vi "cs-scanning_v5_refsonly.vi"() -> ()   [LabVIEW 2017]
uses:
  controls/boolean_info.ctl
  controls/TF-params.ctl
  controls/z-axis-params_v4.ctl
  <vilib>/rvi/Emulation/niFpgaGetClockAttributes.vi
  <vilib>/rvi/Emulation/niFpgaSctlEmulationGetInTimedLoop.vi
  <vilib>/rvi/Emulation/niFpgaEmulationReportErrorSimple.vi
  <vilib>/rvi/Emulation/niFpgaProcessEmulError.vi
  <vilib>/rvi/eio/common/nirviEmuTemplateMethod_errors.vi
  <vilib>/rvi/Emulation/niFpgaEmulationIsFPGAContextNoSignature.vi
  <vilib>/rvi/DataTransferAndStorage/Container/Common/niFpgaContainerGetUniqueNameForEmu.vi
  <vilib>/rvi/Memory/Memory_Emulation/niFpgaMemoryEmulationCacheClearOnFirstRun.vi
  <vilib>/rvi/Memory/Memory_Emulation/nirvimemoryEmulationManagerCache_MakeExclusive.vi
  <vilib>/rvi/Memory/Memory_Emulation/niFpgaMemoryEmulationValidateCache.vi
  <vilib>/rvi/Memory/Memory_Emulation/nirvimemoryEmulationManagerCache_InsertValue.vi
  <vilib>/Utility/error.llb/Clear Errors.vi
  <vilib>/rvi/Memory/Memory_Emulation/nirvimemoryEmulationManagerCache_ReleaseExclusive.vi
  <vilib>/rvi/Memory/Memory_Emulation/nirvimemoryEmulationManagerCache_GetValue.vi
  <vilib>/rvi/Memory/Memory_Emulation/nirvimemoryEmulationManagerCache_SetValue.vi
  <vilib>/rvi/Emulation/niFpgaCriticalErrorInLSC.vi
  <vilib>/eio/EIONode/EIONode.xnode
  <vilib>/rvi/DataTransferAndStorage/Container/XNode/niFpgaContainer.xnode
  <vilib>/rvi/DataTransferAndStorage/Register/Emulation/niFpgaRegisterEmulation.vi
  FPGA-data-logging.lvlib
  libimaging-cs.lvlib
panel:
  in  "scan-rate":fxp<+/-,16,5>
  in  "zup-err-threshold":fxp<+,24,5>=0.10000038146972656 format="%#_21g"
  in  "z_axis_params":T1={"TOL"=0.3, "z_u_max"=5.0, "setpoint-scan"=0.0, "Ki-scan"=0.001, "Z_error_threshold"=0.0, "Z_settled_samples_threshold "=0, "uz_safe"=0.0, "Kiz_down"=0.001, "max_Z_settle_samples"=5000, "setpoint-up"=0.0} {"uz_safe" format="%#_13g"; "Z_error_threshold" format="%#_13g"; "TOL" format="%#_13g"}
  in  "TF-params":T2={"TF-order"=0, "Num"=[0.0, 0.0, 0.0, 0.0, 0.0, 0.0, 0.0, 0.0, 0.0], "Den"=[0.0, 0.0, 0.0, 0.0, 0.0, 0.0, 0.0, 0.0, 0.0]}
  in  "do-Dz":bool
  out "stop_loops":bool
  out "xy_k":fxp<+/-,16,5>[](array[numeric])
  out "xy_ref":fxp<+/-,16,5>[](array[numeric])
  out "u_x saturated":bool
  out "u_y saturated":bool
  out "state1-count":u64
  out "state5-count":u64
  out "state4-count":u64
  out "state3-count":u64
  out "state2-count":u64
  in  "collect all":bool
  out "entity-index":i16
  in  "TsTicks":u32=1600
  out "number-settled-samples-Z":i16
  out "Current Case":u8
  out "boolean \nindicators":T3
  out "z-u(k)":sgl
  in  "ABORT":bool
  out "read fifo timeout":bool
  in  "numEntities":i16
  in  "trigger-0":bool
  out "number-settled-samples-y":i16
  out "number-settled-samples-x":i16
  in  "xy-error-threshold":sgl format="%#_13g"
  in  "settled-samples\nthreshold":i16
  in  "Ki-xy":sgl=0.001 format="%#_13g"
  in  "xy-bound":sgl
  # "- If collect all = fasle ,\nwe only collect measurement data.\n- If collect all = true, we collect everything."
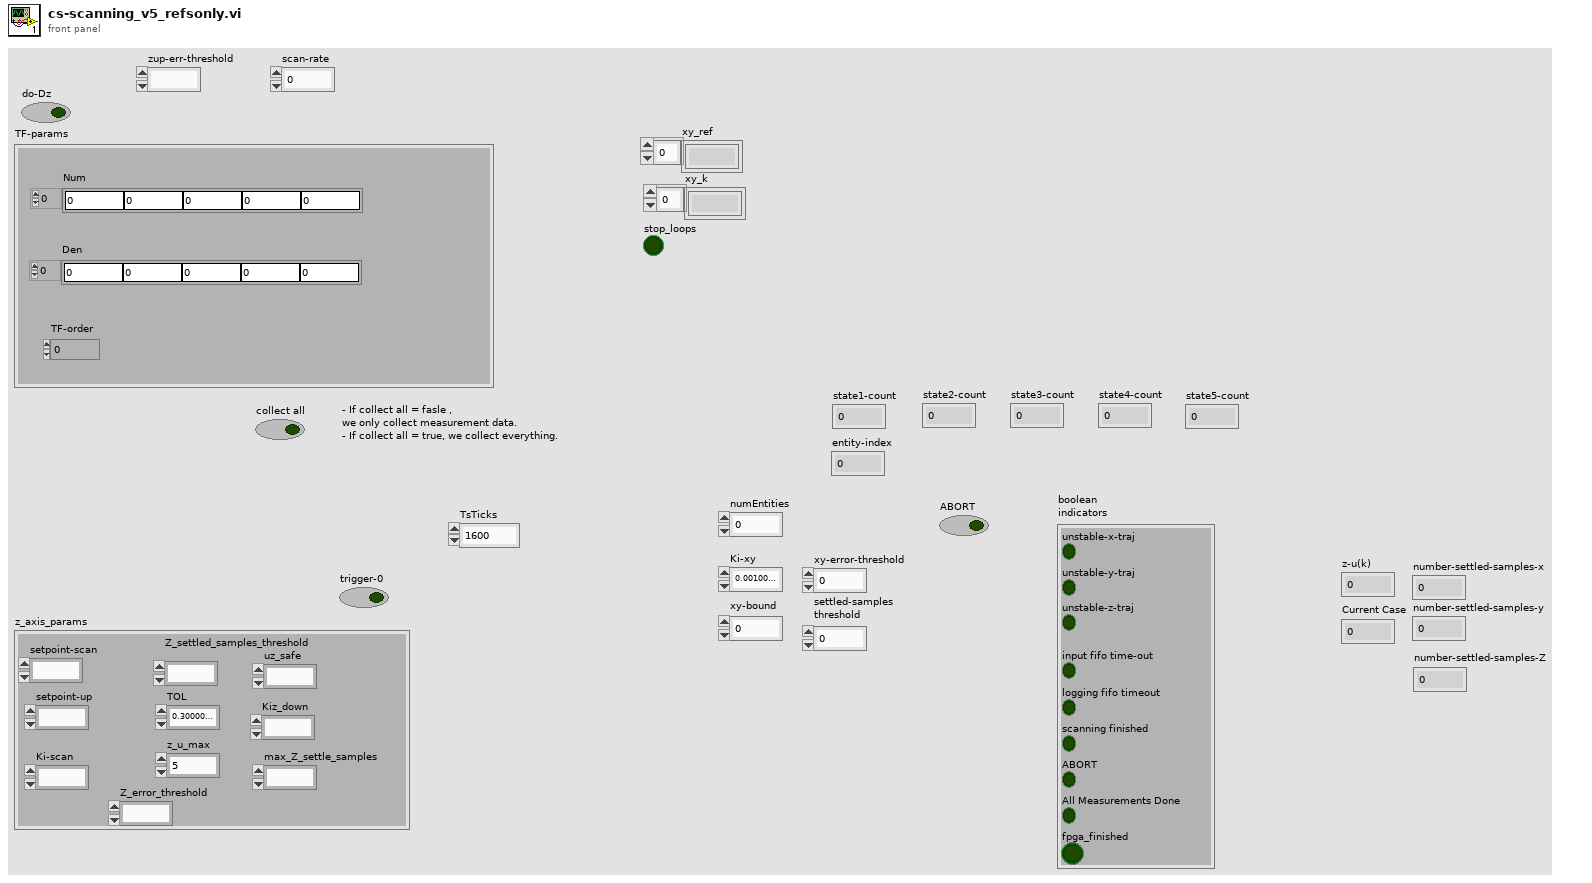
[diagram p1: front panel]
types:
  T1 = typedef "z-axis-params_v4.ctl" = cluster{"TOL":sgl, "z_u_max":sgl, "setpoint-scan":fxp<+/-,32,16>, "Ki-scan":sgl, "Z_error_threshold":sgl, "Z_settled_samples_threshold ":i16, "uz_safe":fxp<+/-,16,5>, "Kiz_down":sgl, "max_Z_settle_samples":i16, "setpoint-up":fxp<+/-,32,16>}
  T2 = typedef "TF-params.ctl" = cluster{"TF-order":i16, "Num":sgl[], "Den":sgl[]}
  T3 = typedef "boolean_info.ctl" = cluster{"unstable-z-traj":bool, "input fifo time-out":bool, "logging fifo timeout":bool, "scanning finished":bool, "unstable-x-traj":bool, "unstable-y-traj":bool, "ABORT":bool, "All Measurements Done":bool, "fpga_finished":bool}
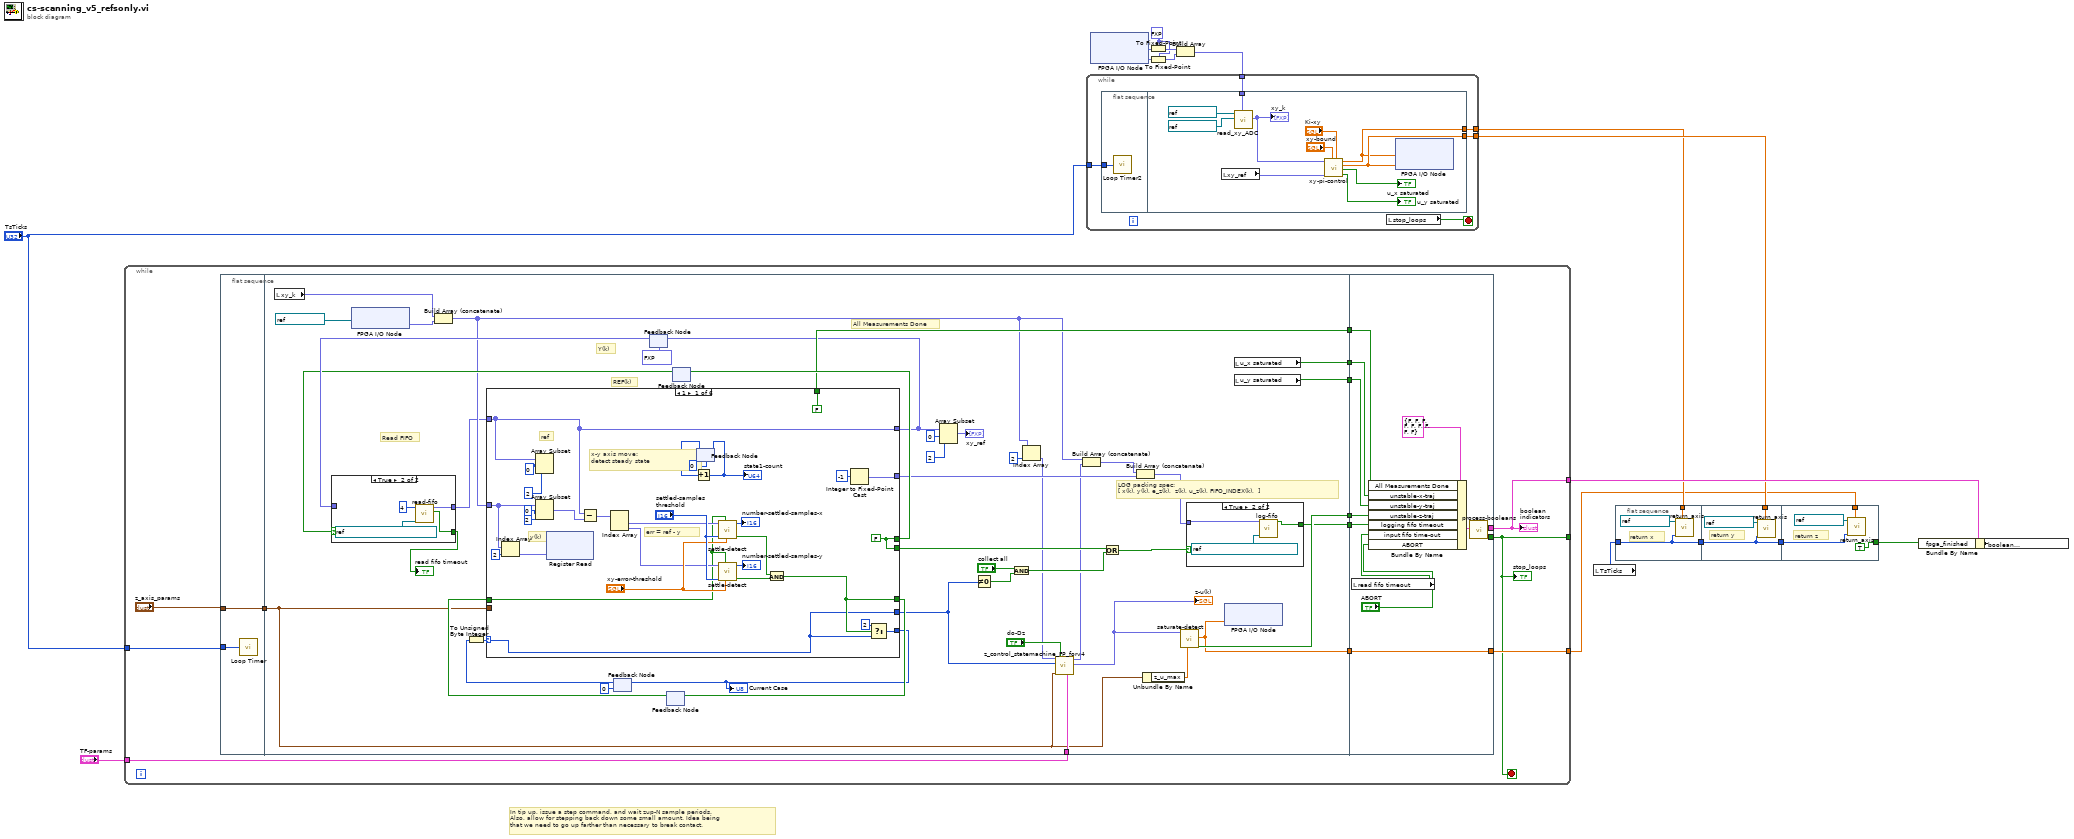
[diagram p0: block diagram]
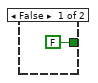
[diagram p2: hidden frame]
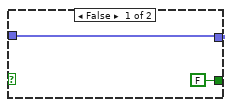
[diagram p3: hidden frame]
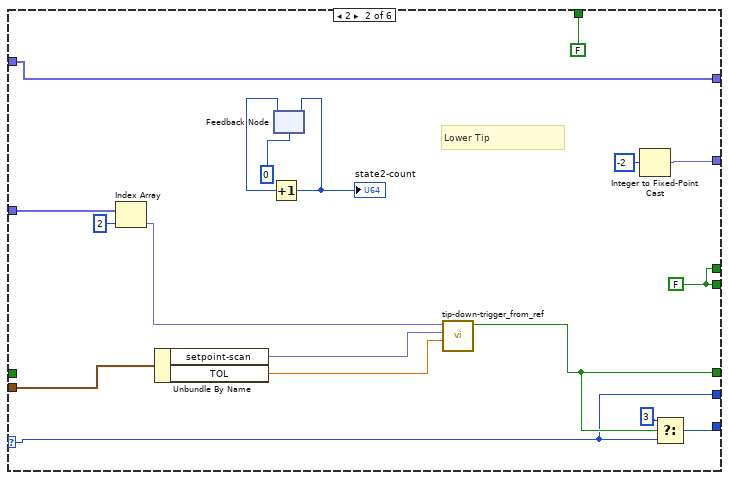
[diagram p4: hidden frame]
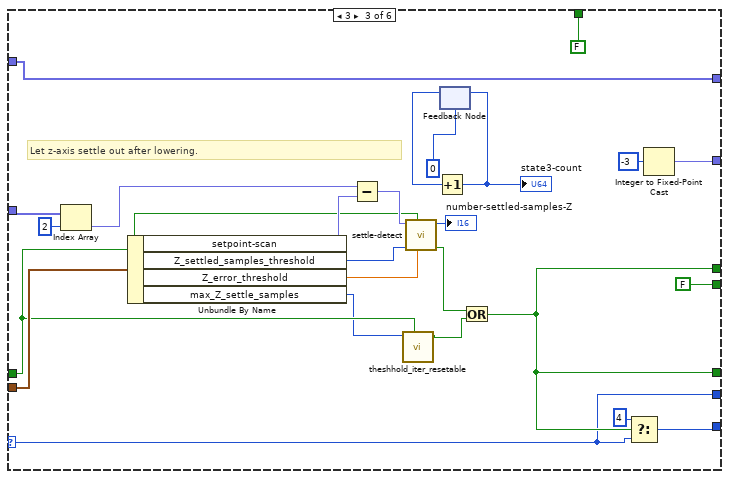
[diagram p5: hidden frame]
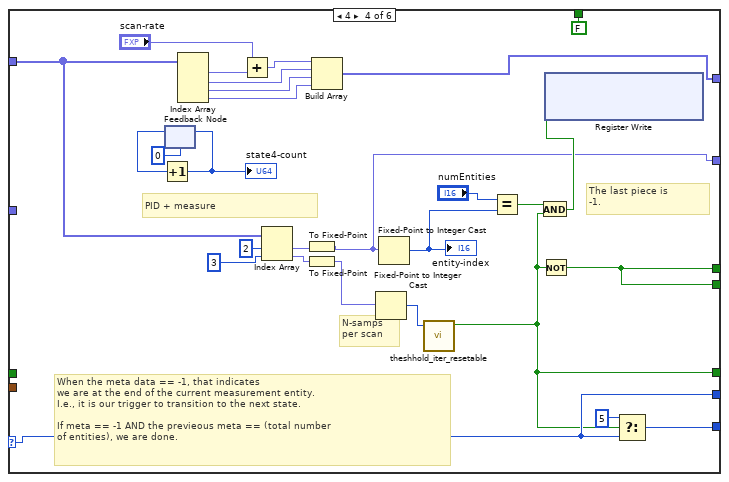
[diagram p6: hidden frame]
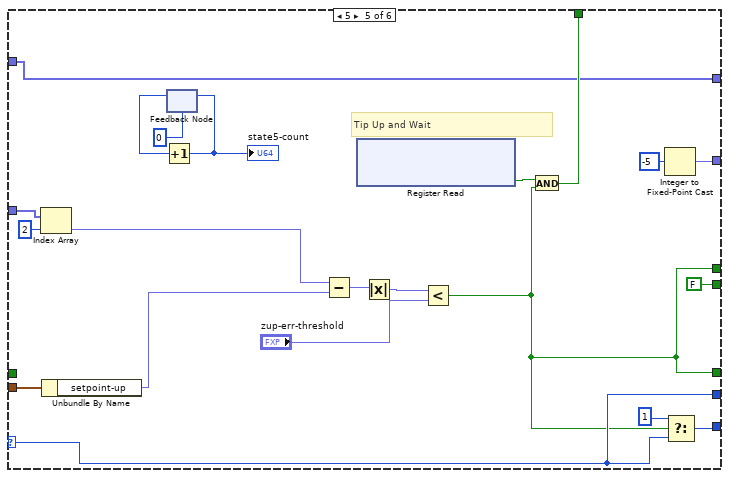
[diagram p7: hidden frame]
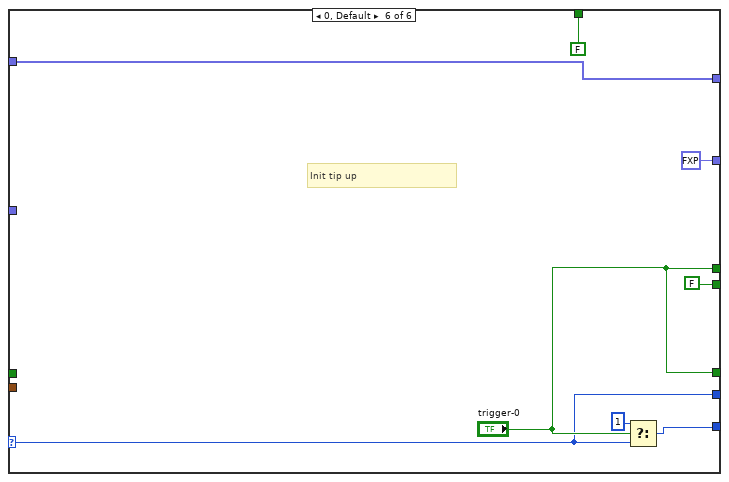
[diagram p8: hidden frame]
diagram:
  w13 = fxp<+/-,16,5> 0.0 ("fixed-point type")
  # "In tip up, issue a step command, and wait zup-N sample periods.\nAlso, allow for stepping back down some small amount. Idea being \nthat we need to go up farther than necessary to break contact."
  n1 = while {
    tunnel: "TsTicks" -> [w26]
    tunnel: [w22] -> _
    tunnel: [w24] -> w2
    tunnel: [w23] -> w9
    tunnel: "TF-params" -> [w19]
    stop <- w22 stop-if-true
    n2 = flat-sequence {
      tunnel: w26 -> [w31]
      tunnel: "z_axis_params" -> [w32]
      tunnel: [w32] -> w30
      tunnel: w30 -> [w36]
      tunnel: [w73] -> w29
      tunnel: [w72] -> w28
      tunnel: [w60] -> w27
      tunnel: [w43] -> w25
      tunnel: [w55] -> w21
      tunnel: [w54] -> w20
      tunnel: w19 -> [w41]
      tunnel: w29 -> [w227]
      tunnel: w28 -> [w224]
      tunnel: w27 -> [w221]
      tunnel: [w220] -> w22
      tunnel: [w219] -> w23
      tunnel: [w218] -> w24
      tunnel: w25 -> [w218]
      tunnel: w21 -> [w217]
      tunnel: w20 -> [w216]
      frame #0 {
        n3 = call "Loop Timer"("Count(Ticks)"=w31) -> ()  [unwired: 1 out]
      }
      frame #1 {
        # "All Measurements Done"
        # "REF(k)"
        # "Y(k)"
        # "LOG packing spec:\n[ x(k), y(k), e_z(k),  z(k), u_z(k), FIFO_INDEX(k),  ]"
        # "Read FIFO"
        n4 = local read "xy_k"() -> (w48:fxp<+/-,16,5>[])
        n5 = xnode "FPGA I/O Node"("FPGA I/O In"=refnum<k21> "Mod2/AI2" ("y - ADC")) -> ("I/O Item"=w52:fxp<+/-,24,5>)  [unwired: 1 out]
        n6 = Build Array (concatenate)(w48, w52) -> (w51:fxp<+/-,24,5>[])
        n7 = feedback #1(u8 0 ("t")) -> (w46:u8)
        n8 = To Unsigned Byte Integer(number=w46) -> (unsigned 8bit integer=w47:u8)
        n9 = feedback #2(fxp<+/-,16,5>[] [0.0, 0.0, 0.0, 0.0] ("unpacked-data")) -> (w75:fxp<+/-,32,5>[])
        n10 = feedback #3() -> (w66:bool)  [unwired: 1 in]
        n11 = feedback #4() -> (w69:bool)  [unwired: 1 in]
        n12 = case shown="True" w69 {
          tunnel: w75 -> [w81 _]
          tunnel: [w81 w83] -> w35
          tunnel: [FALSE ("timout?") w82] -> w71
          frame False {
          }
          frame True {
            n13 = call "read-fifo.vi"("FIFO In"=refnum<k21> "host-to-fpga-fxp-16-5", "numChan"=4) -> ("timout?"=w82:bool, "unpacked-data"=w83:fxp<+/-,16,5>[])  [unwired: 8 in]
          }
        }
        "read fifo timeout" <- w71
        n14 = case shown="1" w47 {
          selector: w47 -> [w87 w119 w136 w175 w195 w209]
          tunnel: [w88 w116 FALSE ("trigger-0") w181 FALSE FALSE] -> w61
          tunnel: [w108 w130 w152 w185 w206 w215] -> w45
          tunnel: w51 -> [w89 w118 w156 _ w197 _]
          tunnel: [w88 w116 w139 w181 w190 "trigger-0"] -> w70
          tunnel: w36 -> [_ w133 w150 _ w189 _]
          tunnel: [FALSE FALSE FALSE FALSE w199 FALSE] -> w60
          tunnel: w66 -> [w99 _ w137 _ _ _]
          tunnel: [w98 w121 w139 w162 w190 "trigger-0"] -> w67
          tunnel: [w92 w122 w142 w160 w200 fxp<+/-,16,5> 0.0 ("Element")] -> w49
          tunnel: [w87 w119 w136 w175 w195 w209] -> w39
          tunnel: w35 -> [w86 w117 w134 w174 w187 w208]
          tunnel: [w86 w117 w134 w168 w187 w208] -> w33
          frame 1 {
            w88 = FALSE
            # "y(k)"
            # "err = ref - y"
            # "ref"
            # "x-y axis move: \ndetect steady state"
            n15 = Index Array(array=w89, index=2) -> (element=w91:fxp<+/-,24,5>)
            n16 = Array Subset(array=w86, index=0, length=2) -> ()  [unwired: 1 out]
            n17 = Array Subset(array=w89, index=0, length=2) -> (w103:fxp<+/-,24,5>[])
            n18 = xnode ("Register Read")("Data"=w91) -> ()  [unwired: 1 in, 1 out]
            n19 = Subtract(x=w86, y=w103) -> (x-y=w97:fxp<+/-,33,6>[])
            n20 = Index Array(array=w97) -> (element #1=w102:fxp<+/-,33,6>, element #2=w101:fxp<+/-,33,6>)  [unwired: 2 in]
            n21 = feedback #5(u64 0) -> (w95:u64)
            n22 = Increment(x=w95) -> (x+1=w96:u64)
            "state1-count" <- w96
            n23 = feedback-in #5(w96) -> ()
            n24 = call "settle-detect.vi"("error-max"="xy-error-threshold", "reset"=w99, "settled-samples\nthreshold"="settled-samples\nthreshold", "err(k)"=w101) -> ("has-settled"=w115:bool, "number-settled-samples"=→"number-settled-samples-y":u16)  [unwired: 6 in]
            n25 = call "settle-detect.vi"("error-max"="xy-error-threshold", "reset"=w99, "settled-samples\nthreshold"="settled-samples\nthreshold", "err(k)"=w102) -> ("has-settled"=w114:bool, "number-settled-samples"=→"number-settled-samples-x":u16)  [unwired: 6 in]
            n26 = And(x=w114, y=w115) -> (x .and. y?=w98:bool)
            n27 = Integer to Fixed-Point Cast(integer=i16 -1) -> (fixed-point=w92:fxp<+/-,16,5>)  [unwired: 1 in]
            n28 = Select(t=u8 2, s=w98, f=w87) -> (s? t:f=w108:u8)
          }
          frame 2 {
            w116 = FALSE
            # "Lower Tip"
            n29 = Index Array(array=w118, index=2) -> (element=w131:fxp<+/-,24,5>)
            n30 = Unbundle By Name(w133) -> ("setpoint-scan"=w123:fxp<+/-,32,16>, "TOL"=w120:sgl)
            n31 = feedback #6(u64 0) -> (w126:u64)
            n32 = Increment(x=w126) -> (x+1=w127:u64)
            "state2-count" <- w127
            n33 = feedback-in #6(w127) -> ()
            n34 = call "tip-down-trigger_from_ref.vi"("TOL"=w120, "setpoint"=w123, "I/O Item"=w131) -> ("Boolean"=w121:bool)  [unwired: 8 in]
            n35 = Integer to Fixed-Point Cast(integer=i16 -2) -> (fixed-point=w122:fxp<+/-,16,5>)  [unwired: 1 in]
            n36 = Select(t=u8 3, s=w121, f=w119) -> (s? t:f=w130:u8)
          }
          frame 3 {
            # "Let z-axis settle out after lowering."
            n37 = Index Array(array=w156, index=2) -> (element=w154:fxp<+/-,24,5>)
            n38 = Unbundle By Name(w150) -> ("setpoint-scan"=w141:fxp<+/-,32,16>, "Z_settled_samples_threshold"=w149:i16, "Z_error_threshold"=w148:sgl, "max_Z_settle_samples"=w135:i16)
            n39 = Subtract(x=w154, y=w141) -> (x-y=w157:fxp<+/-,36,17>)
            n40 = call "theshhold_iter_resetable.vi"("reset"=w137, "N"=w135) -> ("Boolean"=w138:bool)  [unwired: 8 in, 1 out]
            n41 = call "settle-detect.vi"("error-max"=w148, "reset"=w137, "settled-samples\nthreshold"=w149, "err(k)"=w157) -> ("has-settled"=w140:bool, "number-settled-samples"=→"number-settled-samples-Z":u16)  [unwired: 6 in]
            n42 = feedback #7(u64 0) -> (w145:u64)
            n43 = Increment(x=w145) -> (x+1=w146:u64)
            "state3-count" <- w146
            n44 = feedback-in #7(w146) -> ()
            n45 = Or(x=w140, y=w138) -> (x .or. y?=w139:bool)
            n46 = Select(t=u8 4, s=w139, f=w136) -> (s? t:f=w152:u8)
            n47 = Integer to Fixed-Point Cast(integer=i16 -3) -> (fixed-point=w142:fxp<+/-,16,5>)  [unwired: 1 in]
          }
          frame 4 {
            # "N-samps\nper scan"
            # "The last piece is\n-1."
            # "When the meta data == -1, that indicates\nwe are at the end of the current measurement entity.\nI.e., it is our trigger to transition to the next state.\n\nIf meta == -1 AND the previeous meta == (total number\nof entities), we are done."
            # "PID + measure"
            n48 = feedback #8(u64 0) -> (w179:u64)
            n49 = Increment(x=w179) -> (x+1=w180:u64)
            "state4-count" <- w180
            n50 = feedback-in #8(w180) -> ()
            n51 = Index Array(array=w174) -> (element #1=w173:fxp<+/-,32,5>, element #2=w170:fxp<+/-,32,5>, element #3=w169:fxp<+/-,32,5>, element #4=w159:fxp<+/-,32,5>)  [unwired: 4 in]
            n52 = Add(x="scan-rate", y=w173) -> (x+y=w171:fxp<+/-,32,5>)
            n53 = Index Array(array=w174, index #1=2 ("index"), index #2=3 ("index")) -> (element #1=w166:fxp<+/-,32,5>, element #2=w165:fxp<+/-,32,5>)
            n54 = To Fixed-Point(number=w166) -> (fixed-point=w160:fxp<+/-,16,5>)  [unwired: 1 in]
            n55 = To Fixed-Point(number=w165) -> (fixed-point=w164:fxp<+/-,16,5>)  [unwired: 1 in]
            n56 = Build Array(w171, w170, w169, w159) -> (w168:fxp<+/-,32,5>[])
            n57 = Fixed-Point to Integer Cast(1:w164) -> (0:w163:i16)
            n58 = Fixed-Point to Integer Cast(1:w160) -> (0:w161:i16)
            "entity-index" <- w161
            n59 = call "theshhold_iter_resetable.vi"("N"=w163) -> ("Boolean"=w162:bool)  [unwired: 9 in, 1 out]
            n60 = Equal?(x="numEntities", y=w161) -> (x = y?=w182:bool)
            n61 = And(x=w182, y=w162) -> (x .and. y?=w177:bool)
            n62 = Not(x=w162) -> (.not. x?=w181:bool)
            n63 = xnode ("Register Write")("Data"=w177) -> ()  [unwired: 1 in, 1 out]
            n64 = Select(t=u8 5, s=w162, f=w175) -> (s? t:f=w185:u8)
          }
          frame 5 {
            # "Tip Up and Wait"
            n65 = Index Array(array=w197, index=2) -> (element=w194:fxp<+/-,24,5>)
            n66 = Unbundle By Name(w189) -> ("setpoint-up"=w188:fxp<+/-,32,16>)
            n67 = feedback #9(u64 0) -> (w203:u64)
            n68 = Increment(x=w203) -> (x+1=w204:u64)
            "state5-count" <- w204
            n69 = feedback-in #9(w204) -> ()
            n70 = Subtract(x=w194, y=w188) -> (x-y=w193:fxp<+/-,36,17>)
            n71 = xnode ("Register Read")() -> ("Data"=w196:bool)  [unwired: 1 in, 1 out]
            n72 = Absolute Value(x=w193) -> (abs(x)=w192:fxp<+,35,16>)
            n73 = Less?(x=w192, y="zup-err-threshold") -> (x < y?=w190:bool)
            n74 = And(x=w196, y=w190) -> (x .and. y?=w199:bool)
            n75 = Integer to Fixed-Point Cast(integer=i16 -5) -> (fixed-point=w200:fxp<+/-,16,5>)  [unwired: 1 in]
            n76 = Select(t=u8 1, s=w190, f=w195) -> (s? t:f=w206:u8)
          }
          frame 0, Default {
            # "Init tip up"
            n77 = Select(t=u8 1, s="trigger-0", f=w209) -> (s? t:f=w215:u8)
          }
        }
        "Current Case" <- w45
        n78 = feedback-in #1(w45) -> ()
        n79 = feedback-in #2(w33) -> ()
        n80 = feedback-in #3(w67) -> ()
        n81 = feedback-in #4(w70) -> ()
        n82 = Array Subset(array=w33, index=0, length=2) -> (→"xy_ref":fxp<+/-,32,5>[])
        n83 = Not Equal To 0?(x=w39) -> (x != 0?=w64:bool)
        n84 = And(x="collect all", y=w64) -> (x .and. y?=w62:bool)
        n85 = Index Array(array=w51, index=2) -> (element=w38:fxp<+/-,24,5>)
        n86 = call "z_control_statemachine_FP_forv4.vi"("TF-params"=w41, "do-Dz"="do-Dz", "z_axis_params"=w36, "State"=w39, "zerr(k)"=w38) -> ("zuk_Dinv"=w42:fxp<+/-,16,5>, "z-u(k)"=w37:fxp<+/-,16,5>)  [unwired: 5 in]
        "z-u(k)" <- w42
        n87 = Build Array (concatenate)(w51, w37) -> (w50:fxp<+/-,24,5>[])
        n88 = Or(x=w61, y=w62) -> (x .or. y?=w65:bool)
        n89 = Build Array (concatenate)(w50, w49) -> (w74:fxp<+/-,24,5>[])
        n90 = Unbundle By Name(w36) -> ("z_u_max"=w58:sgl)
        n91 = call "saturate-detect.vi"("bound"=w58, "x"=w42) -> ("saturated"=w73:bool, "sat(x)"=w43:sgl)  [unwired: 8 in]
        n92 = case shown="True" w65 {
          tunnel: w74 -> [_ w78]
          tunnel: [FALSE ("logging-timeout?") w77] -> w72
          frame False {
          }
          frame True {
            n93 = call "log-fifo.vi"("FIFO In"=refnum<k21> "fpga-to-host2-fxp-16-5", "input-data"=w78) -> ("logging-timeout?"=w77:bool)  [unwired: 9 in]
          }
        }
        n94 = xnode "FPGA I/O Node"("Mod1/AO2"=w43) -> ()  [unwired: 1 in, 1 out]
        n95 = local read "u_x saturated"() -> (w55:bool)
        n96 = local read "u_y saturated"() -> (w54:bool)
      }
      frame #2 {
        n97 = local read "read fifo timeout"() -> (w223:bool)
        n98 = Bundle By Name(cluster=T3 {"unstable-z-traj"=FALSE, "input fifo time-out"=FALSE, "logging fifo timeout"=FALSE, "scanning finished"=FALSE, "unstable-x-traj"=FALSE, "unstable-y-traj"=FALSE, "ABORT"=FALSE, "All Measurements Done"=FALSE, "fpga_finished"=FALSE} ("boolean errors"), "All Measurements Done"=w221, "unstable-x-traj"=w217, "unstable-y-traj"=w216, "unstable-z-traj"=w227, "logging fifo timeout"=w224, "input fifo time-out"=w223, "ABORT"="ABORT") -> (w225:T3)
        n99 = call "process-booleans.vi"("boolean indicators 2"=w225) -> ("scaning finished"=w220:bool, "boolean indicators"=w219:T3)  [unwired: 9 in]
      }
    }
    "boolean \nindicators" <- w23
    "stop_loops" <- w22
  }
  n100 = xnode "FPGA I/O Node"() -> ("Mod2/AI0"=w16:fxp<+/-,24,5>, "Mod2/AI1"=w14:fxp<+/-,24,5>)  [unwired: 2 in, 2 out]
  n101 = To Fixed-Point(fixed-point type=w13, number=w16) -> (fixed-point=w17:fxp<+/-,16,5>)
  n102 = To Fixed-Point(fixed-point type=w13, number=w14) -> (fixed-point=w15:fxp<+/-,16,5>)
  n103 = Build Array(w17, w15) -> (w3:fxp<+/-,16,5>[])
  n104 = while {
    tunnel: "TsTicks" -> [w232]
    tunnel: [w231] -> w5
    tunnel: [w230] -> w4
    tunnel: w3 -> [w229]
    stop <- w228 stop-if-true
    n105 = flat-sequence {
      tunnel: w232 -> [w233]
      tunnel: [w243] -> w231
      tunnel: [w242] -> w230
      tunnel: w229 -> [w238]
      frame #0 {
        n106 = call "Loop Timer2"("Count(Ticks)"=w233) -> ()  [unwired: 1 out]
      }
      frame #1 {
        n107 = local read "xy_ref"() -> (w235:fxp<+/-,16,5>[])
        n108 = call "read_xy_ADC.vi"("x(0), y(0)"=w238, "y - ADC"=refnum<k21> "Mod2/AI1", "x - ADC"=refnum<k21> "Mod2/AI0") -> ("x_y"=w234:fxp<+/-,17,6>[])  [unwired: 8 in]
        "xy_k" <- w234
        n109 = call "xy-pi-control.vi"("Ki-xy"="Ki-xy", "xy-umax"="xy-bound", "xy-ref"=w235, "x_k-y_k"=w234) -> ("u_y saturated"=→"u_y saturated":bool, "u_x saturated"=→"u_x saturated":bool, "sat(u_y)"=w243:sgl, "sat(u_x)"=w242:sgl)  [unwired: 4 in]
        n110 = xnode "FPGA I/O Node"("Mod1/AO0"=w242, "Mod1/AO1"=w243) -> ()  [unwired: 2 in, 2 out]
      }
    }
    n111 = local read "stop_loops"() -> (w228:bool)
  }
  n112 = local read "TsTicks"() -> (w10:u32)
  n113 = flat-sequence {
    tunnel: w10 -> [w246]
    tunnel: w4 -> [w247]
    tunnel: [w246] -> w12
    tunnel: w5 -> [w250]
    tunnel: w12 -> [w248]
    tunnel: [w248] -> w11
    tunnel: w2 -> [w254]
    tunnel: w11 -> [w252]
    tunnel: [TRUE] -> w8
    frame #0 {
      # "return x"
      n114 = call "return_axis.vi"("u(0)"=w247, "TsTicks"=w246, "FPGA I/O In"=refnum<k21> "Mod1/AO0") -> ()  [unwired: 9 in]
    }
    frame #1 {
      # "return y"
      n115 = call "return_axis.vi"("u(0)"=w250, "TsTicks"=w248, "FPGA I/O In"=refnum<k21> "Mod1/AO1") -> ()  [unwired: 9 in]
    }
    frame #2 {
      # "return z"
      n116 = call "return_axis.vi"("u(0)"=w254, "TsTicks"=w252, "FPGA I/O In"=refnum<k21> "Mod1/AO2") -> ()  [unwired: 9 in]
    }
  }
  n117 = Bundle By Name(cluster=w9, "fpga_finished"=w8) -> (w7:T3)
  n118 = local write "boolean \nindicators"(w7) -> ()
